vi "Field Draw Robot.vi"(0 "Draw Targets?":T1, 4 "IA Judge.Time":enum16{"Azul", "Amarelo"}(ring), 5 "Draw Number":bool, 6 "Robot":T4={"id"=0, "function"=enum."Attacker", "x"=0.0, "y"=0.0, "orientation"=0.0, "v_tangent"=0.0, "v_normal"=0.0, "v_ang"=0.0, "kick_x"=0.0, "kick_z"=0.0, "dribble"=FALSE, "Timestamp"=timestamp(0 s since 1904-01-01), "dest_x"=0.0, "dest_y"=0.0, "dest_orientation"=0.0, "estimatives"={"est_v_tangent"=0.0, "est_v_normal"=0.0, "est_vx"=0.0, "est_vy"=0.0, "Pos Robot Est"=[]}, "dest_x_kick"=0.0, "dest_y_kick"=0.0, "Gap Coord"=[], "States"=enum."GoToTangent"}, 7 "picture in":picture, 8 "color(black)":u32(colorbox)=16775978, 9 "Scale mm/pixel":sgl, 10 "Detection Robot":T7 {"height" format="%+4.3f"; "pixel_y" format="%+4.3f"; "pixel_x" format="%+4.3f"; "orientation" format="%+4.3f"; "y" format="%+4.3f"; "confidence" format="%4.3f"; "x" format="%+4.3f"}, 11 "Offset":T9) -> (3 "picture out":picture)   [LabVIEW 2017]
uses:
  <vilib>/Analysis/NI_AALPro.lvlib
  <vilib>/Analysis/coordinate.llb/2D Cartesian Coordinate Rotation (Scalar).vi
  <vilib>/Utility/miscctls.llb/LVBoundsTypeDef.ctl
  SSL Detection Robot.ctl
  <vilib>/Analysis/Matrix/Datatypes/RealMatrix.ctl
  <vilib>/Analysis/Matrix/NI_Matrix.lvlib
  Core/AI Robot.ctl
  Intel/Functions Enum.ctl
  Intel/AttackerStates.ctl
  DrawTargets.ctl
panel:
  in  "pen Chute":T2={"Width"=3, "Style"=enum."Solid"}
  in  "pen":T3={"Width"=1.0, "Style"=enum."Solid"}
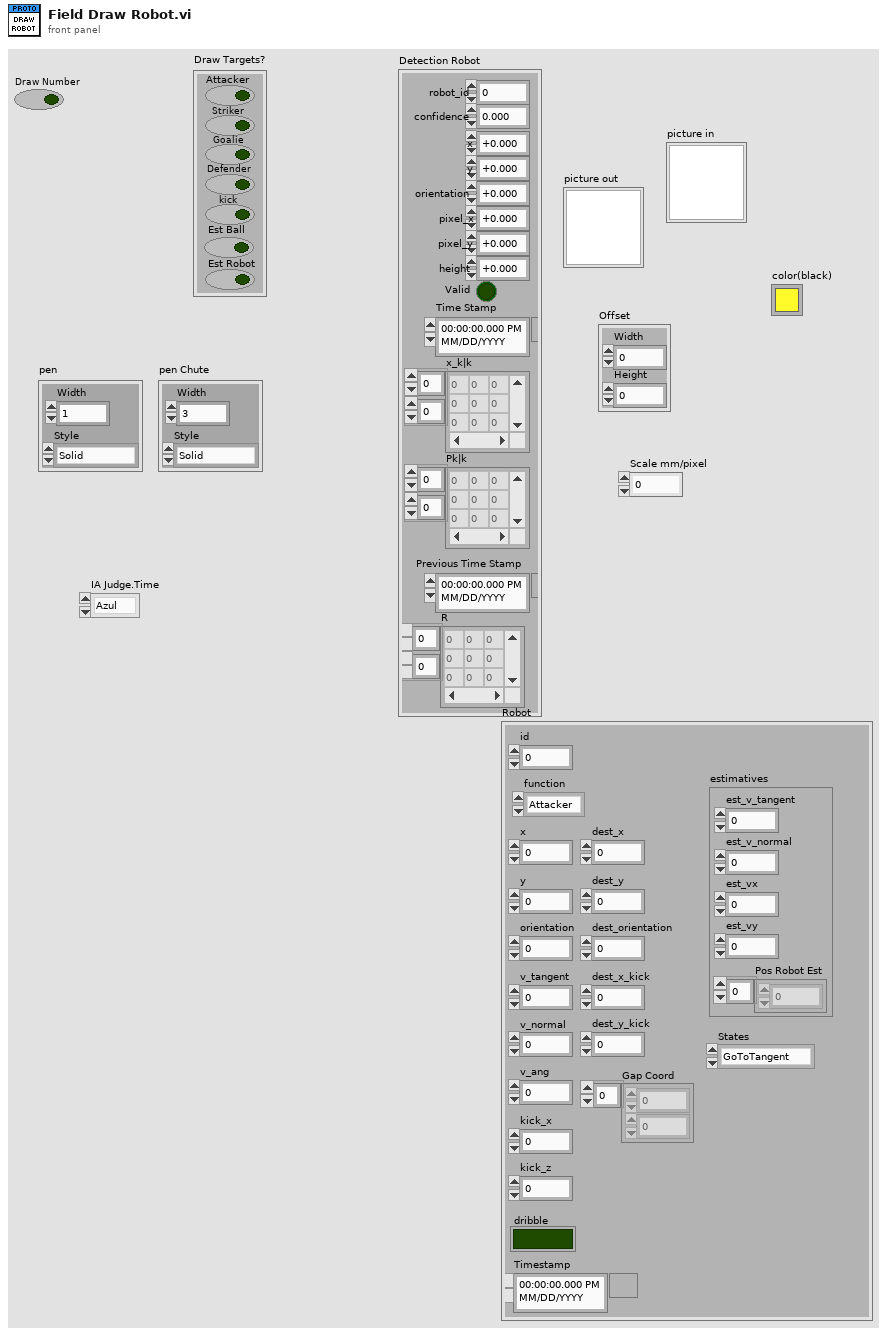
[diagram p1: front panel]
types:
  T1 = typedef "DrawTargets.ctl" = cluster{"Attacker":bool, "Striker":bool, "Goalie":bool, "Defender":bool, "kick":bool, "Est Ball":bool, "Est Robot":bool}
  T2 = cluster{"Width":u16, "Style":enum32{"Solid", "Dash", "Dot", "DashDot", "DashDotDot"}}
  T3 = cluster{"Width":dbl, "Style":enum32{"Solid", "Dash", "Dot", "DashDot", "DashDotDot"}}
  T4 = typedef "AI Robot.ctl" = cluster{"id":u32, "function":T5, "x":dbl, "y":dbl, "orientation":dbl, "v_tangent":dbl, "v_normal":dbl, "v_ang":dbl, "kick_x":dbl, "kick_z":dbl, "dribble":bool, "Timestamp":timestamp, "dest_x":dbl, "dest_y":dbl, "dest_orientation":dbl, "estimatives":cluster{"est_v_tangent":dbl, "est_v_normal":dbl, "est_vx":dbl, "est_vy":dbl, "Pos Robot Est":dbl[]}, "dest_x_kick":dbl, "dest_y_kick":dbl, "Gap Coord":dbl[], "States":T6}
  T5 = typedef "Functions Enum.ctl" = enum16{"Attacker", "Goalie", "Defender", "Striker", "Goto 0", "Dummy", "Kicker", "ZigZag"}
  T6 = typedef "AttackerStates.ctl" = enum16{"Pass", "GoToTangent", "BallGetting", "GoToKick", ""}
  T7 = typedef "SSL Detection Robot.ctl" = cluster{"x":sgl, "robot_id":u32, "confidence":sgl, "y":sgl, "orientation":sgl, "pixel_x":sgl, "pixel_y":sgl, "height":sgl, "Valid":bool, "Time Stamp":timestamp, "x_k|k":T8, "Pk|k":T8, "Previous Time Stamp":timestamp, "R":T8}
  T8 = typedef "NI_Matrix.lvlib/RealMatrix.ctl" = dbl[][]
  T9 = typedef "LVBoundsTypeDef.ctl" = cluster{"Width":u32, "Height":u32}
  T10 = cluster{"horizontal":enum16{"left", "center", "right"}, "vertical":enum16{"top", "center", "bottom"}}
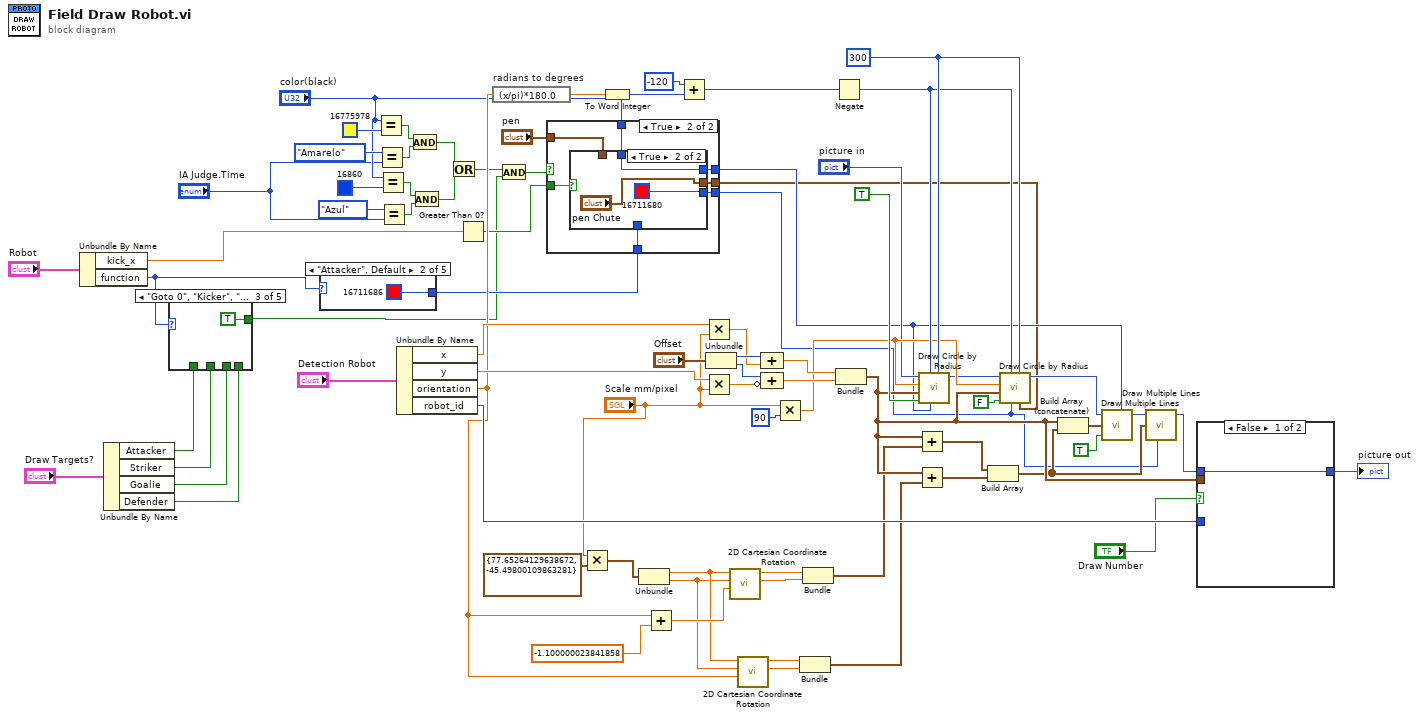
[diagram p0: block diagram]
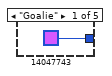
[diagram p8: hidden frame]
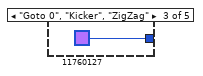
[diagram p9: hidden frame]
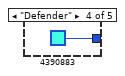
[diagram p10: hidden frame]
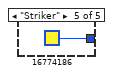
[diagram p11: hidden frame]
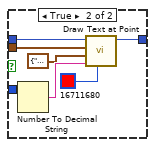
[diagram p12: hidden frame]
diagram:
  w59 = i16 300 ("arc size(360)")
  n1 = Unbundle By Name("Robot") -> ("kick_x"=w29:dbl, "function"=w1:T5)
  n2 = Unbundle By Name("Draw Targets?") -> ("Attacker"=w8:bool, "Striker"=w7:bool, "Goalie"=w6:bool, "Defender"=w5:bool)
  n3 = case shown="\"Goto 0\", \"Kicker\", \"ZigZag\"" w1 {
    tunnel: [w78 w79 TRUE ("Draw Target Striker?") w81 w82] -> w2
    tunnel: w5 -> [_ _ _ w81 _]
    tunnel: w7 -> [_ _ _ _ w82]
    tunnel: w8 -> [w78 _ _ _ _]
    tunnel: w6 -> [_ w79 _ _ _]
    frame "Attacker", Default {
    }
    frame "Goalie" {
    }
    frame "Goto 0", "Kicker", "ZigZag" {
    }
    frame "Defender" {
    }
    frame "Striker" {
    }
  }
  n4 = case shown="\"Attacker\", Default" w1 {
    tunnel: [u32 14047743 ("color(black)") u32 16711686 ("color(black)") u32 11760127 ("color(black)") u32 4390883 ("color(black)") u32 16774186 ("color(black)")] -> w13
    frame "Goalie" {
    }
    frame "Attacker", Default {
    }
    frame "Goto 0", "Kicker", "ZigZag" {
    }
    frame "Defender" {
    }
    frame "Striker" {
    }
  }
  n5 = Equal?(x="color(black)", y=u32 16775978 ("color(black)")) -> (x = y?=w22:bool)
  n6 = Equal?(x=enum16{"Azul", "Amarelo"}."Amarelo", y="IA Judge.Time") -> (x = y?=w23:bool)
  n7 = Equal?(x="color(black)", y=u32 16860 ("color(black)")) -> (x = y?=w19:bool)
  n8 = Equal?(x=enum16{"Azul", "Amarelo"}."Azul", y="IA Judge.Time") -> (x = y?=w20:bool)
  n9 = Unbundle By Name("Detection Robot") -> ("x"=w74:sgl, "y"=w75:sgl, "orientation"=w42:sgl, "robot_id"=w60:u32)
  n10 = And(x=w22, y=w23) -> (x .and. y?=w15:bool)
  n11 = And(x=w19, y=w20) -> (x .and. y?=w14:bool)
  n12 = Or(x=w15, y=w14) -> (x .or. y?=w3:bool)
  n13 = Greater Than 0?(x=w29) -> (x > 0?=w11:bool)
  n14 = expression code="(x/pi)*180.0" "radians to degrees"(w42) -> (w64:sgl)
  n15 = And(x=w3, y=w2) -> (x .and. y?=w4:bool)
  n16 = case shown="True" w4 {
    tunnel: [w89 w96] -> w27
    tunnel: [w89 w95] -> w26
    tunnel: "color(black)" -> [w89 w94]
    tunnel: w13 -> [_ w93]
    tunnel: [w88 w92] -> w12
    tunnel: w11 -> [_ w91]
    tunnel: "pen" -> [w88 w90]
    frame False {
    }
    frame True {
      n17 = case shown="True" w91 {
        tunnel: [w98 u32 16711680 ("color(black)")] -> w95
        tunnel: w94 -> [w99 w101]
        tunnel: [w99 w101] -> w96
        tunnel: w93 -> [w98 _]
        tunnel: [w97 "pen Chute"] -> w92
        tunnel: w90 -> [w97 _]
        frame False {
        }
        frame True {
        }
      }
    }
  }
  n18 = Multiply(x="Scale mm/pixel", y=cluster{sgl, sgl} {77.65264, -45.498} ("appended array")) -> (x*y=w37:cluster{sgl, sgl})
  n19 = To Word Integer(number=w64) -> (16bit integer=w63:i16)
  n20 = Unbundle(w37) -> (w44:sgl, w43:sgl)
  n21 = Add(x=w42, y=sgl -1.1 ("theta")) -> (x+y=w45:sgl)
  n22 = Add(x=i16 -120, y=w63) -> (x+y=w62:i16)
  n23 = Multiply(x=w74, y="Scale mm/pixel") -> (x*y=w70:sgl)
  n24 = Multiply(x=w75, y="Scale mm/pixel") -> (x*y=w67:sgl)
  n25 = Unbundle("Offset") -> ("Width"=w71:u32, "Height"=w68:u32)
  n26 = call-poly <vilib>:"2D Cartesian Coordinate Rotation.vi"("theta"=w45, "y"=w43, "x"=w44) -> ("y out"=w47:dbl, "x out"=w48:dbl)  [unwired: 6 in, 1 out]
  n27 = call-poly <vilib>:"2D Cartesian Coordinate Rotation.vi"("theta"=w42, "y"=w43, "x"=w44) -> ("y out"=w40:dbl, "x out"=w41:dbl)  [unwired: 6 in, 1 out]
  n28 = Compound Arithmetic op=ADD(w71, w70) -> (w69:sgl)
  n29 = Compound Arithmetic op=ADD(w68, invert w67) -> (w66:sgl)
  n30 = Multiply(x="Scale mm/pixel", y=i16 90 ("radius")) -> (x*y=w56:sgl)
  n31 = Bundle("x out"=w41, "y out"=w40) -> (w36:cluster{"x out":dbl, "y out":dbl})  [unwired: 1 in]
  n32 = Bundle("x out"=w48, "y out"=w47) -> (w35:cluster{"x out":dbl, "y out":dbl})  [unwired: 1 in]
  n33 = Negate(x=w62) -> (-x=w58:i16)
  n34 = Bundle(w69, w66) -> (w54:cluster{sgl, sgl})  [unwired: 1 in]
  n35 = Add(x=w54, y=w35) -> (x+y=w33:cluster{dbl, dbl})
  n36 = Add(x=w54, y=w36) -> (x+y=w34:cluster{dbl, dbl})
  n37 = call <vilib>:"Draw Circle by Radius.vi"("arc size(360)"=w59, "color(black)"=w27, "start angle(0)"=w58, "fill?(F)"=TRUE, "pixel center"=w54, "radius"=w56, "picture"="picture in") -> ("new picture"=w30:picture)  [unwired: 4 in]
  n38 = Build Array(w33, w34) -> (w53:cluster{dbl, dbl}[])
  n39 = call <vilib>:"Draw Circle by Radius.vi"("pen"=w12, "arc size(360)"=w59, "color(black)"=w26, "start angle(0)"=w58, "fill?(F)"=FALSE, "pixel center"=w54, "radius"=w56, "picture"=w30) -> ("new picture"=w32:picture)  [unwired: 3 in]
  n40 = Build Array (concatenate)(w54, w53) -> (w51:cluster{dbl, dbl}[])
  n41 = call <vilib>:"Draw Multiple Lines.vi"("picture"=w32, "line endpoints"=w51, "fill?(F)"=TRUE, "color(black)"=w27) -> ("new picture"=w52:picture)  [unwired: 5 in]
  n42 = call <vilib>:"Draw Multiple Lines.vi"("picture"=w52, "line endpoints"=w53, "color(black)"=w26) -> ("new picture"=w55:picture)  [unwired: 6 in]
  n43 = case shown="False" "Draw Number" {
    tunnel: [w103 w110] -> w61
    tunnel: w60 -> [_ w108]
    tunnel: w55 -> [w103 w106]
    tunnel: w54 -> [_ w105]
    frame False {
    }
    frame True {
      n44 = Number To Decimal String(number=w108) -> (decimal integer string=w109:string)  [unwired: 1 in]
      n45 = call <vilib>:"Draw Text at Point.vi"("text color(black)"=u32 16711680, "text"=w109, "alignment(left, top)"=T10 {"horizontal"=enum."center", "vertical"=enum."center"}, "origin"=w105, "picture"=w106) -> ("new picture"=w110:picture)  [unwired: 5 in, 1 out]
    }
  }
  "picture out" <- w61
